vi "VD-getSettings.vi"(8 "error in (no error)":errorcluster, 11 "VD-LV-LiteVNA in":refnum<class "VD-LV-LiteVNA.lvclass">) -> (0 "error out":errorcluster, 2 "Settings status":T1, 3 "VD-LV-LiteVNA out":refnum<class "VD-LV-LiteVNA.lvclass">)   [LabVIEW 2020, in "VD-LV-LiteVNA.lvclass"]
uses:
  VD-LV-LiteVNA.lvclass
  hardware-protocol/serial/HP-S-data.ctl
  VD-settings_status.ctl
  VD-action.ctl
  VD-LV-LiteVNA.lvclass/VD-LV-LiteVNA.ctl
  hardware-protocol/serial/HP-S-Serial.lvclass
panel:
  out "size(s)":i32
  out "read buffer":T2 format="%x"
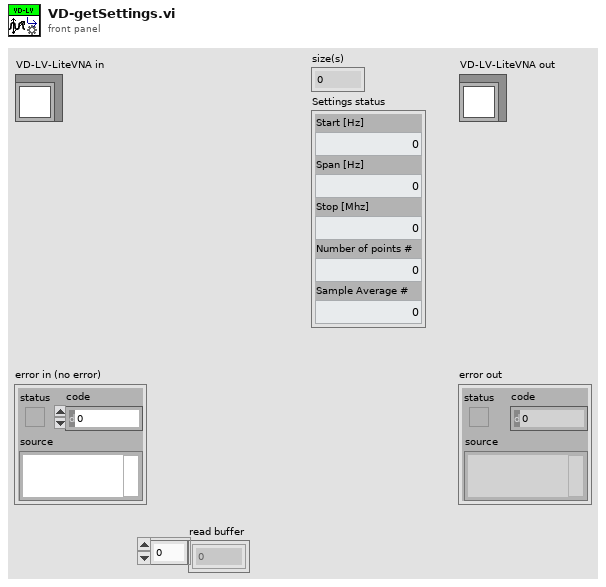
[diagram p1: front panel]
types:
  T1 = typedef "VD-LV-LiteVNA.lvclass/VD-settings_status.ctl" = cluster{"Start [Hz]":u64, "Span [Hz]":u64, "Stop [Mhz]":u64, "Number of points #":u16, "Sample Average #":u16}
  T2 = typedef "HP-S-Serial.lvclass/HP-S-data.ctl" = u8[]
  T3 = typedef "VD-LV-LiteVNA.lvclass/VD-action.ctl" = enum16{"checkCom", "SweepStartHz", "SweepStopHz", "SweepPoints", "valuesPerFrequency", "RawSamplesMode", "ValuesFIFO", "deviceVariant", "protocolVersion", "hardwareRevision", "firmwareMajor", "firmwareMinor"}
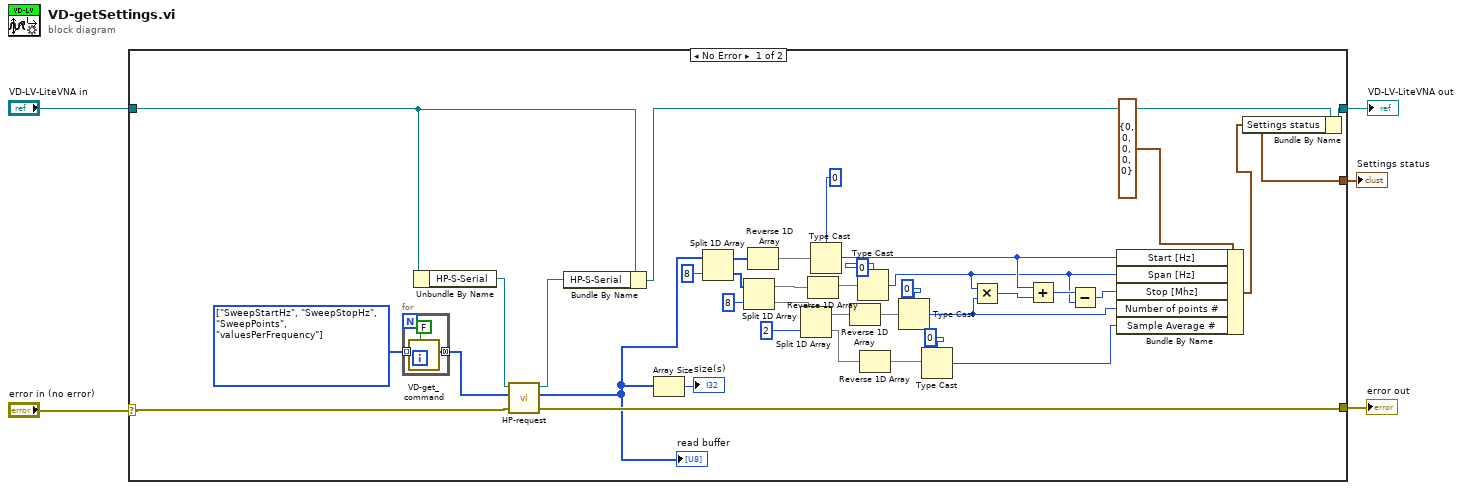
[diagram p0: block diagram]
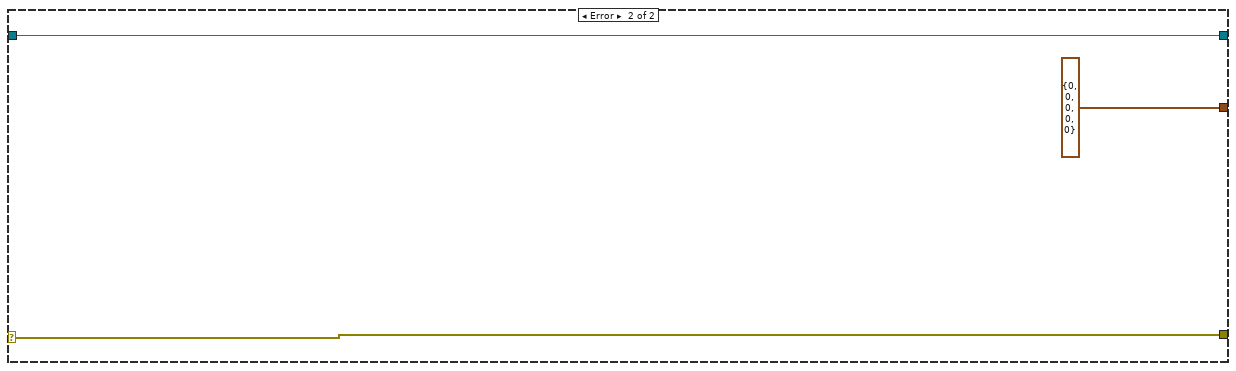
[diagram p2: hidden frame]
diagram:
  n1 = case shown="No Error" "error in (no error)" {
    selector: "error in (no error)" -> [w38 w48]
    tunnel: [w37 w48] -> w4
    tunnel: [w14 w47] -> w2
    tunnel: "VD-LV-LiteVNA in" -> [w36 w47]
    tunnel: [w13 T1 {"Start [Hz]"=0, "Span [Hz]"=0, "Stop [Mhz]"=0, "Number of points #"=0, "Sample Average #"=0} ("Settings status")] -> w1
    frame No Error {
      w39 = T3[] [enum."SweepStartHz", enum."SweepStopHz", enum."SweepPoints", enum."valuesPerFrequency"] items=["checkCom", "SweepStartHz", "SweepStopHz", "SweepPoints", "valuesPerFrequency", "RawSamplesMode", "ValuesFIFO", "deviceVariant", "protocolVersion", "hardwareRevision", "firmwareMajor", "firmwareMinor"] ("Array")
      n2 = for {
        tunnel: [w45] -> w40 mode=concatenating
        tunnel: w39 -> [w44] mode=indexing
        n3 = call "VD-get_command.vi"("Write?"=FALSE, "action"=w44) -> ("Command"=w45:T2)  [unwired: 9 in]
      }
      n4 = Unbundle By Name(w36) -> ("HP-S-Serial"=w42:refnum<class "HP-S-Serial.lvclass">)
      n5 = call-dynamic "HP-request.vi"("error in (no error)"=w38, "write buffer"=w40, "HP-S-Serial in"=w42) -> ("error out"=w37:errorcluster, "read buffer"=w22:T2, "HP-S-Serial out"=w41:refnum<class "HP-S-Serial.lvclass">)  [unwired: 6 in]
      "read buffer" <- w22
      n6 = Bundle By Name(cluster=w36, "HP-S-Serial"=w41) -> (w35:refnum<class "VD-LV-LiteVNA.lvclass">)
      n7 = Array Size(array=w22) -> (size(s)=→"size(s)":i32)
      n8 = Split 1D Array(array=w22, index=8) -> (first subarray=w24:T2, second subarray=w32:T2)
      n9 = Split 1D Array(array=w32, index=8) -> (first subarray=w20:T2, second subarray=w31:T2)
      n10 = Reverse 1D Array(array=w24) -> (reversed array=w23:T2)
      n11 = Split 1D Array(array=w31, index=2) -> (first subarray=w18:T2, second subarray=w16:T2)
      n12 = Reverse 1D Array(array=w20) -> (reversed array=w19:T2)
      n13 = Type Cast(type=u64 0, x=w23) -> (*(type *) &x=w9:u64)
      n14 = Reverse 1D Array(array=w18) -> (reversed array=w17:T2)
      n15 = Type Cast(type=u64 0, x=w19) -> (*(type *) &x=w7:u64)
      n16 = Reverse 1D Array(array=w16) -> (reversed array=w15:T2)
      n17 = Type Cast(type=u16 0, x=w17) -> (*(type *) &x=w11:u16)
      n18 = Type Cast(type=u16 0, x=w15) -> (*(type *) &x=w25:u16)
      n19 = Multiply(x=w7, y=w11) -> (x*y=w10:u64)
      n20 = Add(x=w9, y=w10) -> (x+y=w8:u64)
      n21 = Subtract(x=w8, y=w7) -> (x-y=w6:u64)
      n22 = Bundle By Name(cluster=T1 {"Start [Hz]"=0, "Span [Hz]"=0, "Stop [Mhz]"=0, "Number of points #"=0, "Sample Average #"=0} ("Settings status"), "Start [Hz]"=w9, "Span [Hz]"=w7, "Stop [Mhz]"=w6, "Number of points #"=w11, "Sample Average #"=w25) -> (w13:T1)
      n23 = Bundle By Name(cluster=w35, "Settings status"=w13) -> (w14:refnum<class "VD-LV-LiteVNA.lvclass">)
    }
    frame Error {
    }
  }
  "error out" <- w4
  "VD-LV-LiteVNA out" <- w2
  "Settings status" <- w1
